vi "PickUpBallAuto.vi"(8 "error in (no error)":errorcluster) -> ()   [LabVIEW 2015]
uses:
  Utilities/VisionGlobals.vi
  Utilities/MotorPositionGlobals.vi
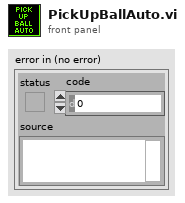
[diagram p1: front panel]
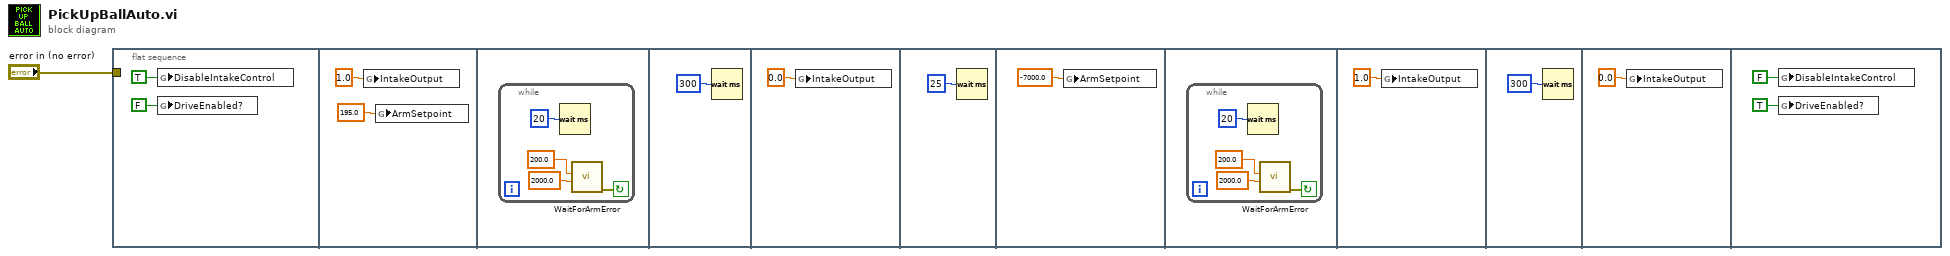
[diagram p0: block diagram]
diagram:
  n1 = flat-sequence {
    tunnel: "error in (no error)" -> [_]
    frame #0 {
      n2 = global write "MotorPositionGlobals.vi" "DisableIntakeControl"(TRUE ("DisableIntakeControl")) -> ()
      n3 = global write "VisionGlobals.vi" "DriveEnabled?"(FALSE ("DriveEnabled?")) -> ()
    }
    frame #1 {
      n4 = global write "MotorPositionGlobals.vi" "IntakeOutput"(1.0 ("IntakeOutput")) -> ()
      n5 = global write "MotorPositionGlobals.vi" "ArmSetpoint"(195.0 ("ArmSetpoint")) -> ()
    }
    frame #2 {
      n6 = while {
        stop <- w7 continue-if-true
        n7 = Wait (ms)(milliseconds to wait=u32 20) -> ()  [unwired: 1 out]
        n8 = call "WaitForArmError.vi"("Timeout (ms)"=2000.0, "AllowedError"=200.0) -> ("error out"=w7:errorcluster)  [unwired: 9 in]
      }
    }
    frame #3 {
      n9 = Wait (ms)(milliseconds to wait=u32 300) -> ()  [unwired: 1 out]
    }
    frame #4 {
      n10 = global write "MotorPositionGlobals.vi" "IntakeOutput"(0.0 ("IntakeOutput")) -> ()
    }
    frame #5 {
      n11 = Wait (ms)(milliseconds to wait=u32 25) -> ()  [unwired: 1 out]
    }
    frame #6 {
      n12 = global write "MotorPositionGlobals.vi" "ArmSetpoint"(-7000.0 ("ArmSetpoint")) -> ()
    }
    frame #7 {
      n13 = while {
        stop <- w15 continue-if-true
        n14 = Wait (ms)(milliseconds to wait=u32 20) -> ()  [unwired: 1 out]
        n15 = call "WaitForArmError.vi"("Timeout (ms)"=2000.0, "AllowedError"=200.0) -> ("error out"=w15:errorcluster)  [unwired: 9 in]
      }
    }
    frame #8 {
      n16 = global write "MotorPositionGlobals.vi" "IntakeOutput"(1.0 ("IntakeOutput")) -> ()
    }
    frame #9 {
      n17 = Wait (ms)(milliseconds to wait=u32 300) -> ()  [unwired: 1 out]
    }
    frame #10 {
      n18 = global write "MotorPositionGlobals.vi" "IntakeOutput"(0.0 ("IntakeOutput")) -> ()
    }
    frame #11 {
      n19 = global write "MotorPositionGlobals.vi" "DisableIntakeControl"(FALSE ("DisableIntakeControl")) -> ()
      n20 = global write "VisionGlobals.vi" "DriveEnabled?"(TRUE ("DriveEnabled?")) -> ()
    }
  }
